vi "AllThingsBaxter_ROS.vi"   [LabVIEW 2010]
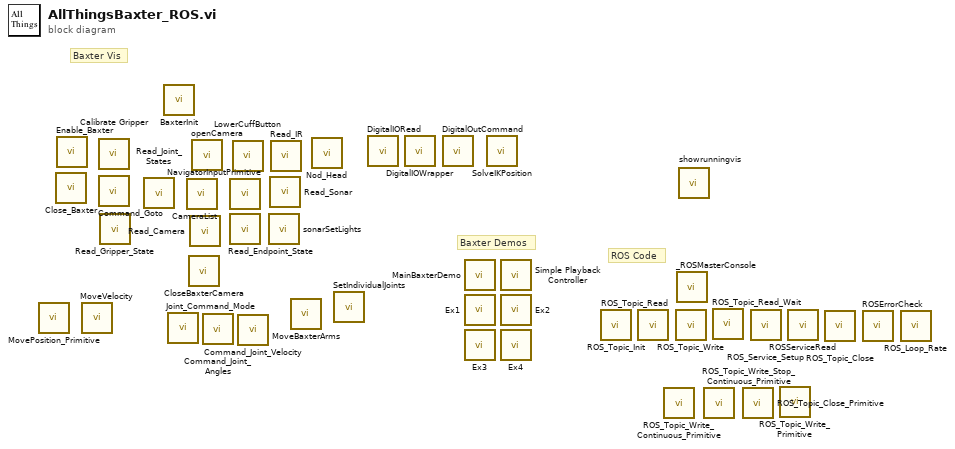
[diagram p0: block diagram]
diagram:
  # "ROS Code"
  # "Baxter Demos"
  # "Baxter Vis"
  n1 = call <userlib>:"MovePosition_Primitive.vi"() -> ()  [unwired: 6 in, 1 out]
  n2 = call <userlib>:"Close_Baxter.vi"() -> ()  [unwired: 4 in, 1 out]
  n3 = call <userlib>:"Enable_Baxter.vi"() -> ()  [unwired: 4 in, 1 out]
  n4 = call <userlib>:"MoveVelocity.vi"() -> ()  [unwired: 7 in, 1 out]
  n5 = call <userlib>:"Calibrate Gripper.vi"() -> ()  [unwired: 6 in, 1 out]
  n6 = call <userlib>:"Command_Goto.vi"() -> ()  [unwired: 6 in, 1 out]
  n7 = call <userlib>:"Read_Gripper_State.vi"() -> ()  [unwired: 3 in, 2 out]
  n8 = call <userlib>:"Read_Joint_States.vi"() -> ()  [unwired: 3 in, 2 out]
  n9 = call <userlib>:"BaxterInit.vi"() -> ()  [unwired: 12 in]
  n10 = call <userlib>:"Joint_Command_Mode.vi"() -> ()  [unwired: 6 in, 1 out]
  n11 = call <userlib>:"CameraList.vi"() -> ()  [unwired: 2 in, 2 out]
  n12 = call <userlib>:"CloseBaxterCamera.vi"() -> ()  [unwired: 3 in, 3 out]
  n13 = call <userlib>:"Read_Camera.vi"() -> ()  [unwired: 3 in, 2 out]
  n14 = call <userlib>:"openCamera.vi"() -> ()  [unwired: 3 in, 2 out]
  n15 = call <userlib>:"Command_Joint_Angles.vi"() -> ()  [unwired: 6 in, 1 out]
  n16 = call <userlib>:"NavigatorInputPrimitive.vi"() -> ()  [unwired: 3 in, 2 out]
  n17 = call <userlib>:"Read_Endpoint_State.vi"() -> ()  [unwired: 3 in, 2 out]
  n18 = call <userlib>:"LowerCuffButton.vi"() -> ()  [unwired: 3 in, 2 out]
  n19 = call <userlib>:"Command_Joint_Velocity.vi"() -> ()  [unwired: 6 in, 1 out]
  n20 = call <userlib>:"sonarSetLights.vi"() -> ()  [unwired: 4 in, 1 out]
  n21 = call <userlib>:"Read_Sonar.vi"() -> ()  [unwired: 3 in, 2 out]
  n22 = call <userlib>:"Read_IR.vi"() -> ()  [unwired: 3 in, 2 out]
  n23 = call <userlib>:"MoveBaxterArms.vi"() -> ()  [unwired: 6 in, 1 out]
  n24 = call <userlib>:"Nod_Head.vi"() -> ()  [unwired: 4 in, 1 out]
  n25 = call <userlib>:"SetIndividualJoints.vi"() -> ()  [unwired: 6 in, 1 out]
  n26 = call <userlib>:"DigitalIORead.vi"() -> ()  [unwired: 4 in, 2 out]
  n27 = call <userlib>:"DigitalIOWrapper.vi"() -> ()  [unwired: 3 in, 2 out]
  n28 = call <userlib>:"DigitalOutCommand.vi"() -> ()  [unwired: 5 in, 1 out]
  n29 = call <userlib>:"MainBaxterDemo.vi"() -> ()  [unwired: 12 in]
  n30 = call <userlib>:"Ex1.vi"() -> ()  [unwired: 12 in]
  n31 = call <userlib>:"Ex3.vi"() -> ()  [unwired: 12 in]
  n32 = call <userlib>:"SolveIKPosition.vi"() -> ()  [unwired: 7 in, 1 out]
  n33 = call <userlib>:"Simple Playback Controller.vi"() -> ()  [unwired: 12 in]
  n34 = call <userlib>:"Ex2.vi"() -> ()  [unwired: 12 in]
  n35 = call <userlib>:"Ex4.vi"() -> ()  [unwired: 12 in]
  n36 = call <userlib>:"ROS_Topic_Init.vi"() -> ()  [unwired: 3 in, 1 out]
  n37 = call <userlib>:"ROS_Topic_Read.vi"() -> ()  [unwired: 2 in, 2 out]
  n38 = call <userlib>:"ROS_Topic_Write_Continuous_Primitive.vi"() -> ()  [unwired: 3 in, 1 out]
  n39 = call <userlib>:"ROS_Topic_Write.vi"() -> ()  [unwired: 4 in, 1 out]
  n40 = call <userlib>:"_ROSMasterConsole.vi"() -> ()  [unwired: 12 in]
  n41 = call <userlib>:"showrunningvis.vi"() -> ()  [unwired: 1 in]
  n42 = call <userlib>:"ROS_Topic_Write_Stop_Continuous_Primitive.vi"() -> ()  [unwired: 12 in]
  n43 = call <userlib>:"ROS_Topic_Read_Wait.vi"() -> ()  [unwired: 2 in, 2 out]
  n44 = call <userlib>:"ROS_Topic_Close_Primitive.vi"() -> ()  [unwired: 3 in, 1 out]
  n45 = call <userlib>:"ROS_Service_Setup.vi"() -> ()  [unwired: 3 in, 3 out]
  n46 = call <userlib>:"ROS_Topic_Write_Primitive.vi"() -> ()  [unwired: 3 in, 1 out]
  n47 = call <userlib>:"ROSServiceRead.vi"() -> ()  [unwired: 2 in, 3 out]
  n48 = call <userlib>:"ROS_Topic_Close.vi"() -> ()  [unwired: 4 in, 1 out]
  n49 = call <userlib>:"ROSErrorCheck.vi"() -> ()  [unwired: 3 in, 1 out]
  n50 = call <userlib>:"ROS_Loop_Rate.vi"() -> ()  [unwired: 5 in, 2 out]
